vi "determine_pixel_coordinates_of_position.vi"(7 "pixel positions":T2, 8 "error in (no error)":errorcluster, 10 "pixel position":T1, 11 "Image in":refnum<class "Image.lvclass">) -> (0 "error out":errorcluster, 2 "Point Coordinates":cluster{"X":dbl, "Y":dbl}, 3 "Image out":refnum<class "Image.lvclass">)   [LabVIEW 2010, in "Image.lvclass"]
uses:
  Image.lvclass
  pixel_positions_cluster.ctl
  pixel_position_cluster.ctl
  Image.lvclass/Image.ctl
  ErrorController/ErrorController/class_data.vi
  ErrorController/ErrorController/ErrorController.lvclass
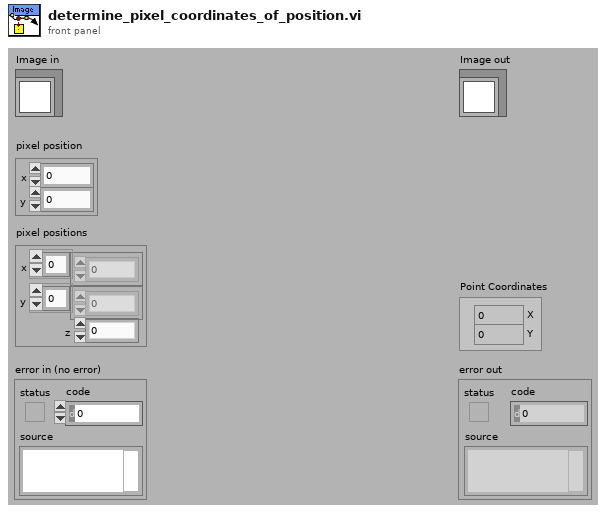
[diagram p1: front panel]
types:
  T1 = typedef "Image.lvclass/pixel_position_cluster.ctl" = cluster{"x":dbl, "y":dbl}
  T2 = typedef "Image.lvclass/pixel_positions_cluster.ctl" = cluster{"x":dbl[], "y":dbl[], "z":dbl}
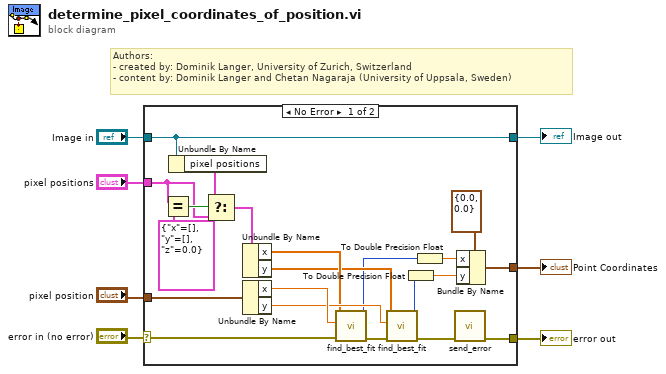
[diagram p0: block diagram]
diagram:
  # "Authors: \n- created by: Dominik Langer, University of Zurich, Switzerland\n- content by: Dominik Langer and Chetan Nagaraja (University of Uppsala, Sweden)"
  n1 = case shown="No Error" "error in (no error)" {
    selector: "error in (no error)" -> [w25 w30]
    tunnel: "pixel position" -> [w26 _]
    tunnel: [w8 w30] -> w6
    tunnel: [w27 _] -> w7
    tunnel: "Image in" -> [w13 w29]
    tunnel: [w13 w29] -> w3
    tunnel: "pixel positions" -> [w12 _]
    frame No Error {
      n2 = Equal?(x=w12, y=T2 {"x"=[], "y"=[], "z"=0.0} ("pixel positions")) -> (x = y?=w14:bool)
      n3 = Unbundle By Name(w13) -> ("pixel positions"=w11:T2)
      n4 = Select(t=w11, s=w14, f=w12) -> (s? t:f=w10:T2)
      n5 = Unbundle By Name(w10) -> ("x"=w22:dbl[], "y"=w21:dbl[])
      n6 = Unbundle By Name(w26) -> ("x"=w24:dbl, "y"=w23:dbl)
      n7 = call "find_best_fit.vi"("error in (no error)"=w25, "value to be found"=w24, "search space"=w22) -> ("error out"=w28:errorcluster, "index of best match"=w19:i32)  [unwired: 6 in, 1 out]
      n8 = call "find_best_fit.vi"("error in (no error)"=w28, "value to be found"=w23, "search space"=w21) -> ("error out"=w9:errorcluster, "index of best match"=w17:i32)  [unwired: 6 in, 1 out]
      n9 = To Double Precision Float(number=w17) -> (double precision float=w16:dbl)
      n10 = To Double Precision Float(number=w19) -> (double precision float=w18:dbl)
      n11 = call "send_error.vi"("error in (no error)"=w9) -> ("error out"=w8:errorcluster)  [unwired: 10 in]
      n12 = Bundle By Name(cluster=cluster{"x":dbl, "y":dbl} {"x"=0.0, "y"=0.0} ("input cluster"), "x"=w18, "y"=w16) -> (w27:cluster{"x":dbl, "y":dbl})
    }
    frame Error {
    }
  }
  "error out" <- w6
  "Image out" <- w3
  "Point Coordinates" <- w7
